vi "plotCSVLabview.vi"() -> ()   [LabVIEW 2018]
uses:
  <vilib>/Utility/file.llb/Read From Spreadsheet File (DBL).vi
panel:
  in  "?":path
  in  "?":path
  in  "?":path
  in  "?":path
  out "Waveform Graph":dbl[][](graph)
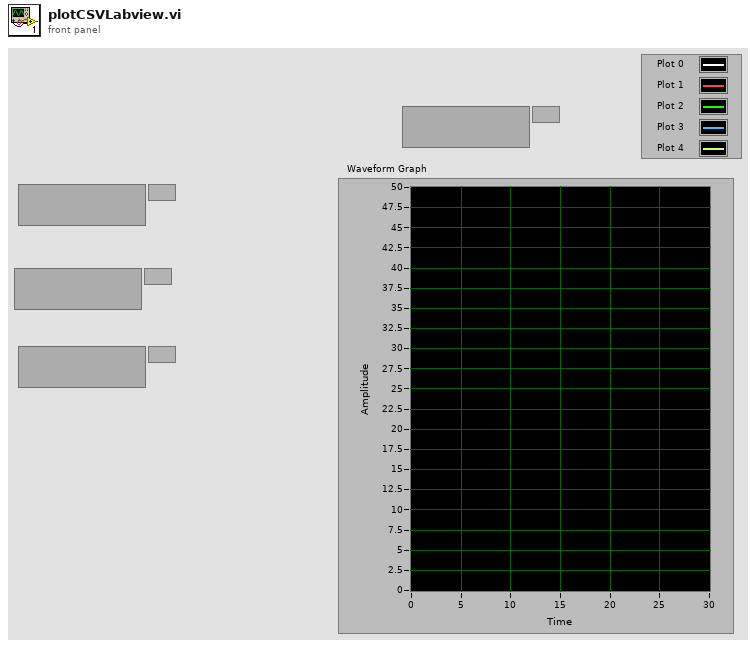
[diagram p1: front panel]
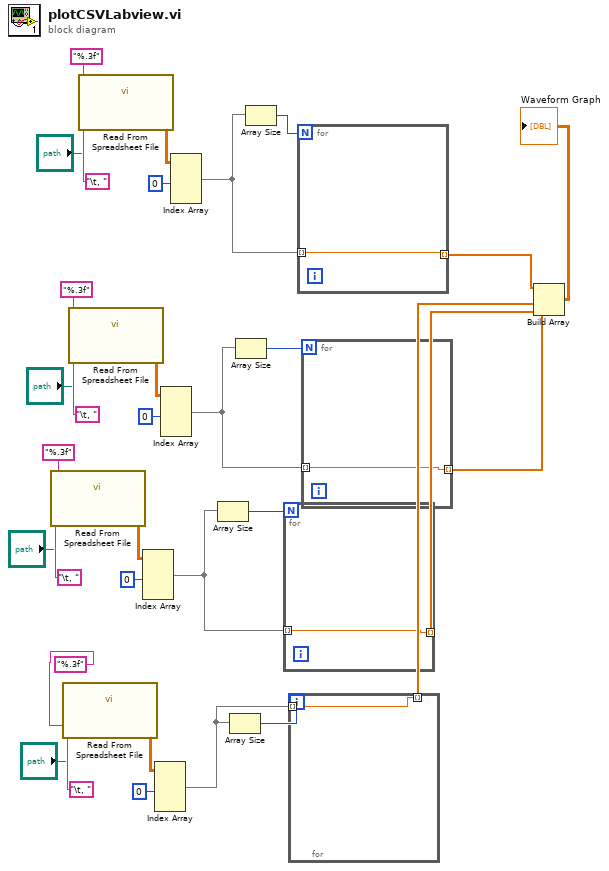
[diagram p0: block diagram]
diagram:
  n1 = call-poly <vilib>:"Read From Spreadsheet File.vi"("delimiter (\\t)"="\t, " ("delimiter (\\t)"), "format (%.3f)"="%.3f", "file path (dialog if empty)"="?") -> ("all rows"=w11:dbl[][])  [unwired: 4 in, 4 out]
  n2 = call-poly <vilib>:"Read From Spreadsheet File.vi"("delimiter (\\t)"="\t, " ("delimiter (\\t)"), "format (%.3f)"="%.3f", "file path (dialog if empty)"="?") -> ("all rows"=w5:dbl[][])  [unwired: 4 in, 4 out]
  n3 = call-poly <vilib>:"Read From Spreadsheet File.vi"("delimiter (\\t)"="\t, " ("delimiter (\\t)"), "format (%.3f)"="%.3f", "file path (dialog if empty)"="?") -> ("all rows"=w21:dbl[][])  [unwired: 4 in, 4 out]
  n4 = call-poly <vilib>:"Read From Spreadsheet File.vi"("delimiter (\\t)"="\t, " ("delimiter (\\t)"), "format (%.3f)"="%.3f", "file path (dialog if empty)"="?") -> ("all rows"=w17:dbl[][])  [unwired: 4 in, 4 out]
  n5 = Index Array(array=w11, index (col) #1=0 ("disabled index (col)")) -> (element #1=w13:dbl[])  [unwired: 3 in, 1 out]
  n6 = Index Array(array=w5, index (col) #1=0 ("disabled index (col)")) -> (element #1=w7:dbl[])  [unwired: 3 in, 1 out]
  n7 = Index Array(array=w21, index (col) #1=0 ("disabled index (col)")) -> (element #1=w23:dbl[])  [unwired: 3 in, 1 out]
  n8 = Index Array(array=w17, index (col) #1=0 ("disabled index (col)")) -> (element #1=w29:dbl[])  [unwired: 3 in, 1 out]
  n9 = Array Size(array=w13) -> (size(s)=w16:i32)
  n10 = Array Size(array=w7) -> (size(s)=w10:i32)
  n11 = Array Size(array=w23) -> (size(s)=w26:i32)
  n12 = Array Size(array=w29) -> (size(s)=w32:i32)
  n13 = for {
    N: w16 -> [_]
    tunnel: [w34] -> w2 mode=indexing
    tunnel: w13 -> [w34] mode=indexing
  }
  n14 = for {
    N: w10 -> [_]
    tunnel: [w35] -> w1 mode=indexing
    tunnel: w7 -> [w35] mode=indexing
  }
  n15 = for {
    N: w32 -> [_]
    tunnel: [w36] -> w19 mode=indexing
    tunnel: w29 -> [w36] mode=indexing
  }
  n16 = for {
    N: w26 -> [_]
    tunnel: [w37] -> w18 mode=indexing
    tunnel: w23 -> [w37] mode=indexing
  }
  n17 = Build Array(w19, w18, w1, w2) -> (→"Waveform Graph":dbl[][])
